vi "getTaskChannel.vi"(8 "error in (no error)":errorcluster, 11 "ExampleTask_MsgUserEventStopNotifier In":refnum<class "Task_MsgUserEventStopMech.lvclass">) -> (0 "error out":errorcluster, 2 "taskChannel":refnum<class "ITaskChannel.lvclass">, 3 "ExampleTask_MsgUserEventStopNotifier Out":refnum<class "Task_MsgUserEventStopMech.lvclass">)   [LabVIEW 2023, in "Task_MsgUserEventStopMech.lvclass"]
doc: "Returns the Task Channel type used by the task."
uses:
  Task_MsgUserEventStopMech.lvclass
  ITaskChannel/ITaskChannel.lvclass
  MsgUETaskChannel/MsgUETaskChannel.lvclass
  C:/projects/TLC_Daemon/source/ITaskChannel/ITaskChannel.lvclass
  MsgUETaskChannel/MsgUETaskChannel.lvclass/MsgUETaskChannel.ctl
  MsgUETaskChannel/Write stopMessage.vi
  Task_MsgUserEventStopMech.lvclass/Task_MsgUserEventStopMech.ctl
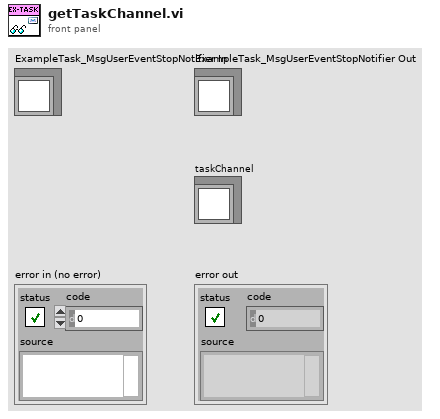
[diagram p1: front panel]
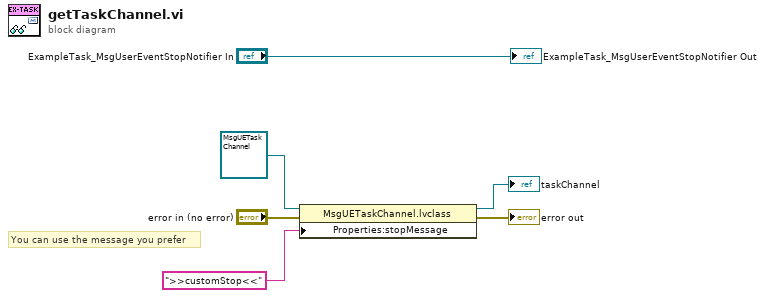
[diagram p0: block diagram]
diagram:
  # "You can use the message you prefer"
  n1 = property class="MsgUETaskChannel.lvclass"(reference=refnum<class "MsgUETaskChannel.lvclass"> refnum ("TLC_Daemon.lvlib:MsgUETaskChannel.lvclass"), error in="error in (no error)", "Properties:stopMessage"=">>customStop<<" ("stopMessage")) -> (reference out=→"taskChannel":refnum<class "MsgUETaskChannel.lvclass">, error out=→"error out":errorcluster)
  "ExampleTask_MsgUserEventStopNotifier Out" <- "ExampleTask_MsgUserEventStopNotifier In"
